vi "34970_CRISTALIZADOR Module.vi"(5 "Agilent 34970A":bool=TRUE, 6 "Freq(T)/Total":bool=TRUE, 7 "Command":T2, 8 "error in (no error)":errorcluster, 10 "Canales":T1={"CH PT100"=["201", "202", "205", "210"], "CH TcK"=["208"], "CH Qhz"=["208"]}, 11 "VISA Agilent 34970A":refnum<visa-resource-name>="COM42") -> (0 "error out":errorcluster, 1 "Qhz":dbl[](array[numeric]), 2 "TcK":dbl[](array[numeric]), 3 "PT100":dbl[](array[numeric]))   [LabVIEW 2017]
uses:
  34970_CRISTALIZADOR Module.ctl
  34970_Canales.ctl
  <instrlib>/Agilent 34970/Agilent 34970.lvlib
panel:
  # "Input Data"
  # "Output Data"
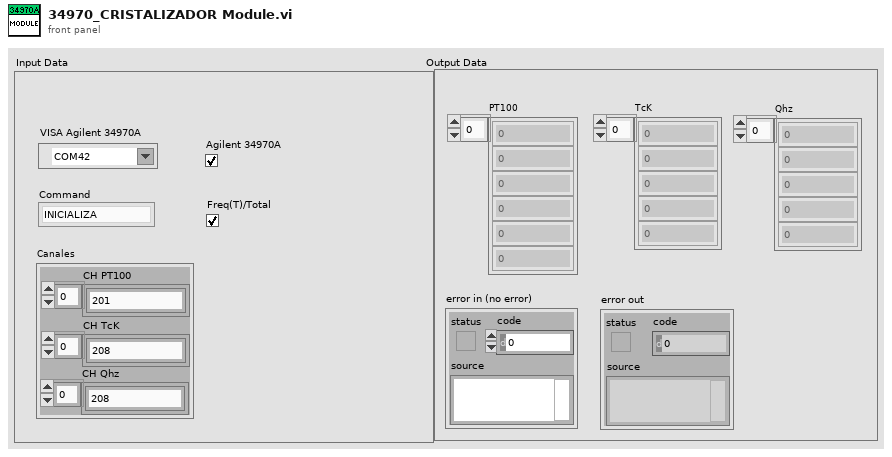
[diagram p1: front panel]
types:
  T1 = typedef "34970_Canales.ctl" = cluster{"CH PT100":string[], "CH TcK":string[], "CH Qhz":string[]}
  T2 = typedef "34970_CRISTALIZADOR Module.ctl" = enum16{"INICIALIZA", "CONFIGURA CANALES", "LECTURA PT100", "LECTURA TERMOPAR", "LECTURA CAUDAL", "LECTURA VOLTAJE", "LECTURA CORRIENTE", "SHUTDOWN"}
  T3 = cluster{"Timeout Value (10000)":u32, "Baud Rate (57600)":enum16{"1200", "2400", "4800", "9600", "19200", "38400", "57600", "115200"}, "Flow Control (1:XON/XOFF)":enum16{"None", "XON / XOFF", "RTS / CTS", "DTR / DSR"}}
  T4 = enum16{"Thermocouple", "Thermistor", "RTD", "4-Wire RTD", "Default (Last)"}
  T5 = enum16{"B", "E", "J", "K", "N", "R", "S", "T", "Default (Last)"}
  T6 = enum16{"100 mV", "1 V", "10 V", "100 V", "300 V", "Auto", "Minimum", "Maximum"}
  T7 = enum16{"4 1/2", "5 1/2", "6 1/2", "Least", "Highest", "Default"}
  T8 = enum16{"10 mA", "100 mA", "1 A", "Auto", "Minimum", "Maximum"}
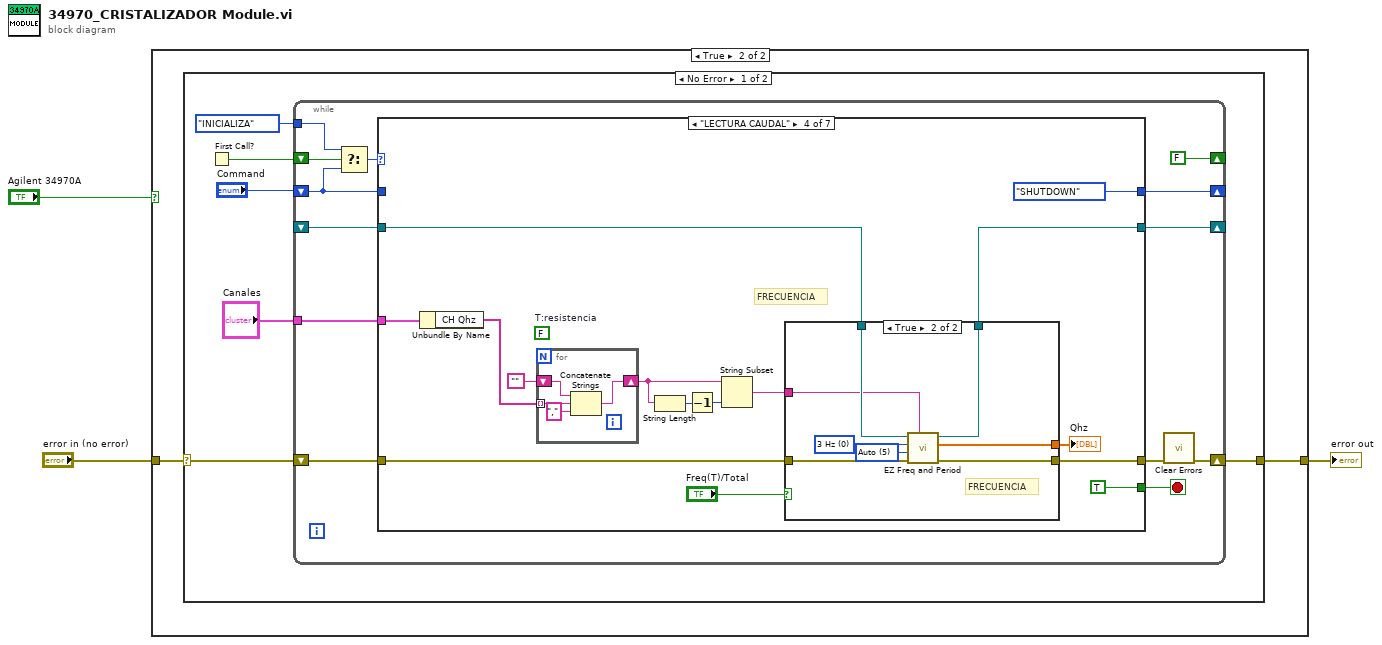
[diagram p0: block diagram]
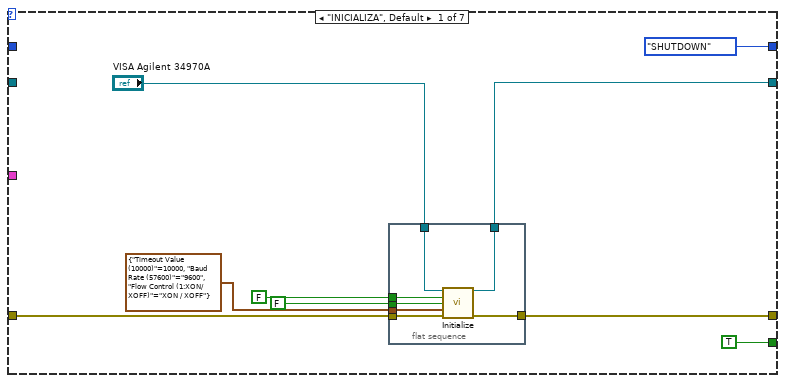
[diagram p3: hidden frame]
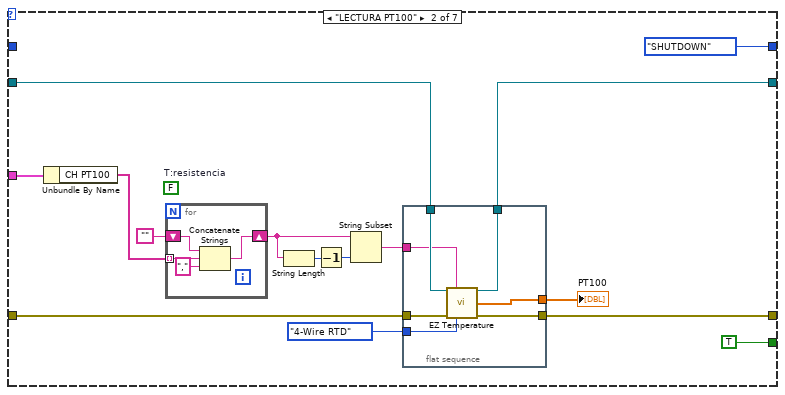
[diagram p4: hidden frame]
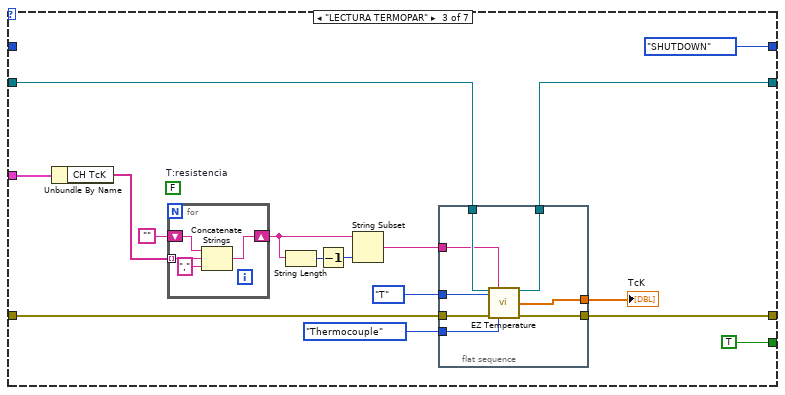
[diagram p5: hidden frame]
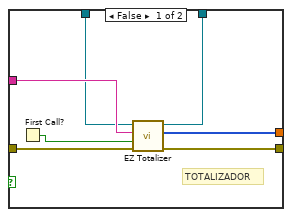
[diagram p6: hidden frame]
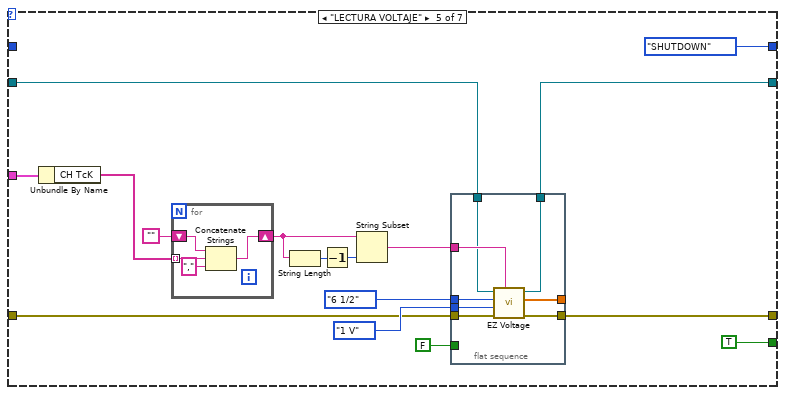
[diagram p7: hidden frame]
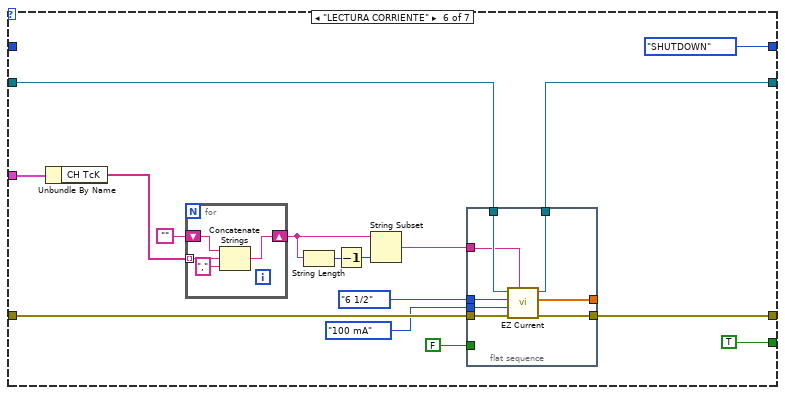
[diagram p8: hidden frame]
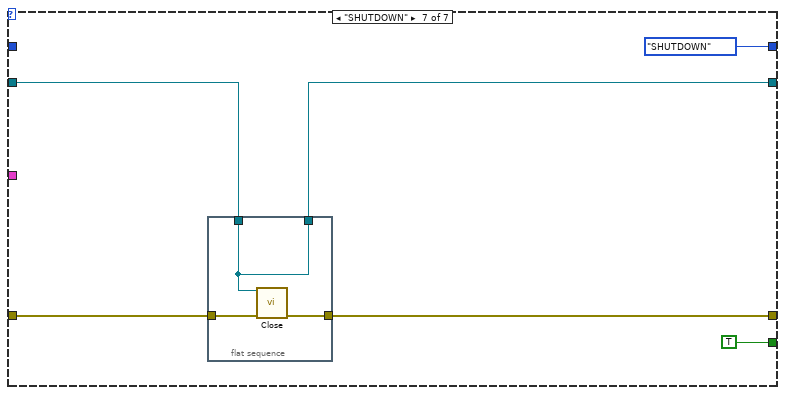
[diagram p9: hidden frame]
diagram:
  n1 = case shown="True" "Agilent 34970A" {
    tunnel: "error in (no error)" -> [w4 w6]
    tunnel: [w4 w5] -> w2
    frame False {
    }
    frame True {
      n2 = case shown="No Error" w6 {
        selector: w6 -> [w10 w195]
        tunnel: [w9 w195] -> w5
        frame No Error {
          n3 = First Call?() -> (First Call?: T/F=w12:bool)
          n4 = while {
            shift-right: [w19] -> _
            shift-left: "Command" -> [w20]
            shift-right: [w13] -> w9
            shift-left: w10 -> [w22]
            shift-right: [FALSE ("First Call?: T/F")] -> _
            shift-left: w12 -> [w25]
            tunnel: 34970_CRISTALIZADOR_Module."INICIALIZA" ("t") -> [w24]
            shift-right: [w17] -> _
            shift-left: _ -> [w18]
            tunnel: "Canales" -> [w15]
            stop <- w23 stop-if-true
            n5 = Select(t=w24, s=w25, f=w20) -> (s? t:f=w16:T2)
            n6 = case shown="\"LECTURA CAUDAL\"" w16 {
              tunnel: [TRUE TRUE TRUE TRUE TRUE TRUE TRUE] -> w23
              tunnel: w22 -> [w31 w53 w80 w107 w133 w163 w191]
              tunnel: w20 -> [_ _ _ _ _ _ _]
              tunnel: [34970_CRISTALIZADOR_Module."SHUTDOWN" ("t") 34970_CRISTALIZADOR_Module."SHUTDOWN" ("t") 34970_CRISTALIZADOR_Module."SHUTDOWN" ("t") 34970_CRISTALIZADOR_Module."SHUTDOWN" ("t") 34970_CRISTALIZADOR_Module."SHUTDOWN" ("t") 34970_CRISTALIZADOR_Module."SHUTDOWN" ("t") 34970_CRISTALIZADOR_Module."SHUTDOWN" ("t")] -> w19
              tunnel: [w30 w47 w74 w101 w142 w170 w190] -> w14
              tunnel: w18 -> [_ w54 w81 w108 w132 w162 w187]
              tunnel: [w29 w46 w73 w100 w143 w171 w186] -> w17
              tunnel: w15 -> [_ w44 w72 w99 w131 w159 _]
              frame "INICIALIZA", Default {
                n7 = flat-sequence {
                  tunnel: "VISA Agilent 34970A" -> [w40]
                  tunnel: w31 -> [w39]
                  tunnel: [w38] -> w30
                  tunnel: [w41] -> w29
                  tunnel: T3 {"Timeout Value (10000)"=10000, "Baud Rate (57600)"=enum."9600", "Flow Control (1:XON/XOFF)"=enum."XON / XOFF"} ("Serial Port Configuration") -> [w37]
                  tunnel: FALSE ("Reset (T: Reset)") -> [w36]
                  tunnel: FALSE ("ID Query (T: Check)") -> [w35]
                  frame #0 {
                    n8 = call <instrlib>:"Initialize.vi"("VISA Resource Name"=w40, "ID Query (T: Check)"=w35, "Reset (T: Reset)"=w36, "Serial Port Configuration"=w37, "error in (no error)"=w39) -> ("VISA Resource Name Out"=w41:refnum<visa-resource-name>, "error out"=w38:errorcluster)  [unwired: 9 in]
                  }
                }
              }
              frame "LECTURA PT100" {
                (unwired) FALSE  # T:resistencia
                n9 = Unbundle By Name(w44) -> ("CH PT100"=w43:string[])
                n10 = for {
                  tunnel: w43 -> [w66] mode=indexing
                  shift-right: [w65] -> w52
                  shift-left: "" -> [w67]
                  n11 = Concatenate Strings(w67, w66, "," ("string")) -> (w65:string)
                }
                n12 = String Length(string=w52) -> (length=w50:i32)
                n13 = Decrement(x=w50) -> (x-1=w51:i32)
                n14 = String Subset(string=w52, length (rest)=w51) -> (substring=w48:string)  [unwired: 1 in]
                n15 = flat-sequence {
                  tunnel: w54 -> [w63]
                  tunnel: w53 -> [w59]
                  tunnel: w48 -> [w57]
                  tunnel: [w61] -> w47
                  tunnel: [w62] -> w46
                  tunnel: [w60] -> w45
                  tunnel: T4."4-Wire RTD" ("Transducer Type (4:Def-Last)") -> [w58]
                  frame #0 {
                    n16 = call <instrlib>:"EZ Temperature.vi"("VISA Resource Name"=w63, "Scan List (empty)"=w57, "error in (no error)"=w59, "Transducer Type (4:Def-Last)"=w58) -> ("VISA Resource Name Out"=w62:refnum<visa-resource-name>, "Output Array"=w60:dbl[], "error out"=w61:errorcluster)  [unwired: 9 in]
                  }
                }
                "PT100" <- w45
              }
              frame "LECTURA TERMOPAR" {
                (unwired) FALSE  # T:resistencia
                n17 = Unbundle By Name(w72) -> ("CH TcK"=w71:string[])
                n18 = for {
                  tunnel: w71 -> [w94] mode=indexing
                  shift-right: [w93] -> w79
                  shift-left: "" -> [w95]
                  n19 = Concatenate Strings(w95, w94, "," ("string")) -> (w93:string)
                }
                n20 = String Length(string=w79) -> (length=w77:i32)
                n21 = Decrement(x=w77) -> (x-1=w78:i32)
                n22 = String Subset(string=w79, length (rest)=w78) -> (substring=w75:string)  [unwired: 1 in]
                n23 = flat-sequence {
                  tunnel: w81 -> [w91]
                  tunnel: w80 -> [w87]
                  tunnel: w75 -> [w85]
                  tunnel: [w89] -> w74
                  tunnel: [w90] -> w73
                  tunnel: [w88] -> w69
                  tunnel: T4."Thermocouple" ("Transducer Type (4:Def-Last)") -> [w86]
                  tunnel: T5."T" ("Thermocouple Type (8:Def-Last)") -> [w84]
                  frame #0 {
                    n24 = call <instrlib>:"EZ Temperature.vi"("VISA Resource Name"=w91, "Scan List (empty)"=w85, "Thermocouple Type (8:Def-Last)"=w84, "error in (no error)"=w87, "Transducer Type (4:Def-Last)"=w86) -> ("VISA Resource Name Out"=w90:refnum<visa-resource-name>, "Output Array"=w88:dbl[], "error out"=w89:errorcluster)  [unwired: 8 in]
                  }
                }
                "TcK" <- w69
              }
              frame "LECTURA CAUDAL" {
                (unwired) FALSE  # T:resistencia
                # "FRECUENCIA"
                n25 = Unbundle By Name(w99) -> ("CH Qhz"=w98:string[])
                n26 = for {
                  tunnel: w98 -> [w128] mode=indexing
                  shift-right: [w127] -> w106
                  shift-left: "" -> [w129]
                  n27 = Concatenate Strings(w129, w128, "," ("string")) -> (w127:string)
                }
                n28 = String Length(string=w106) -> (length=w104:i32)
                n29 = Decrement(x=w104) -> (x-1=w105:i32)
                n30 = String Subset(string=w106, length (rest)=w105) -> (substring=w102:string)  [unwired: 1 in]
                n31 = case shown="True" "Freq(T)/Total" {
                  tunnel: w108 -> [w114 w125]
                  tunnel: w107 -> [w117 w124]
                  tunnel: w102 -> [w116 w123]
                  tunnel: [w113 w122] -> w101
                  tunnel: [w115 w121] -> w100
                  tunnel: [w112 w120] -> w97
                  frame False {
                    # "TOTALIZADOR"
                    n32 = First Call?() -> (First Call?: T/F=w111:bool)
                    n33 = call <instrlib>:"EZ Totalizer.vi"("error in (no error)"=w117, "Read/R-Reset (F:Read)"=w111, "Scan List (empty)"=w116, "VISA Resource Name"=w114) -> ("error out"=w113:errorcluster, "Output Array"=w112:u32[], "VISA Resource Name Out"=w115:refnum<visa-resource-name>)  [unwired: 5 in]
                  }
                  frame True {
                    w118 = u16 5 items=["100 mV", "1 V", "10 V", "100 V", "300 V", "Auto", "Minimum", "Maximum"] ("Range (5:Auto)")
                    w119 = u16 0 items=["3 Hz", "20 Hz", "200 Hz", "MIN", "MAX"] ("Low Frequency (1: 20 Hz)")
                    # "FRECUENCIA"
                    n34 = call <instrlib>:"EZ Freq and Period.vi"("Scan List (empty)"=w123, "error in (no error)"=w124, "Range (5:Auto)"=w118, "Low Frequency (1: 20 Hz)"=w119, "VISA Resource Name"=w125) -> ("error out"=w122:errorcluster, "Output Array"=w120:dbl[], "VISA Resource Name Out"=w121:refnum<visa-resource-name>)  [unwired: 4 in]
                  }
                }
                "Qhz" <- w97
              }
              frame "LECTURA VOLTAJE" {
                n35 = Unbundle By Name(w131) -> ("CH TcK"=w130:string[])
                n36 = for {
                  tunnel: w130 -> [w156] mode=indexing
                  shift-right: [w155] -> w141
                  shift-left: "" -> [w157]
                  n37 = Concatenate Strings(w157, w156, "," ("string")) -> (w155:string)
                }
                n38 = String Length(string=w141) -> (length=w139:i32)
                n39 = Decrement(x=w139) -> (x-1=w140:i32)
                n40 = String Subset(string=w141, length (rest)=w140) -> (substring=w134:string)  [unwired: 1 in]
                n41 = flat-sequence {
                  tunnel: [w146] -> w143
                  tunnel: [w150] -> w142
                  tunnel: FALSE ("AC/DC (F:DC)") -> [_]
                  tunnel: T7."6 1/2" ("Resolution (5:Default)") -> [w147]
                  tunnel: T6."1 V" ("Range (5:Auto)") -> [w148]
                  tunnel: w134 -> [w153]
                  tunnel: w133 -> [w149]
                  tunnel: w132 -> [w152]
                  tunnel: [w151] -> _
                  frame #0 {
                    n42 = call <instrlib>:"EZ Voltage.vi"("Scan List (empty)"=w153, "error in (no error)"=w149, "Range (5:Auto)"=w148, "Resolution (5:Default)"=w147, "VISA Resource Name"=w152) -> ("error out"=w150:errorcluster, "Output Array"=w151:dbl[], "VISA Resource Name Out"=w146:refnum<visa-resource-name>)  [unwired: 4 in]
                  }
                }
              }
              frame "LECTURA CORRIENTE" {
                n43 = Unbundle By Name(w159) -> ("CH TcK"=w158:string[])
                n44 = for {
                  tunnel: w158 -> [w184] mode=indexing
                  shift-right: [w183] -> w169
                  shift-left: "" -> [w185]
                  n45 = Concatenate Strings(w185, w184, "," ("string")) -> (w183:string)
                }
                n46 = String Length(string=w169) -> (length=w167:i32)
                n47 = Decrement(x=w167) -> (x-1=w168:i32)
                n48 = String Subset(string=w169, length (rest)=w168) -> (substring=w164:string)  [unwired: 1 in]
                n49 = flat-sequence {
                  tunnel: [w180] -> w171
                  tunnel: [w178] -> w170
                  tunnel: FALSE ("AC/DC (F:DC)") -> [_]
                  tunnel: w164 -> [w174]
                  tunnel: w163 -> [w179]
                  tunnel: w162 -> [w181]
                  tunnel: T7."6 1/2" ("Resolution (3:Least)") -> [w176]
                  tunnel: T8."100 mA" ("Range (3:Auto)") -> [w175]
                  tunnel: [w177] -> _
                  frame #0 {
                    n50 = call <instrlib>:"EZ Current.vi"("Scan List (empty)"=w174, "error in (no error)"=w179, "Range (3:Auto)"=w175, "Resolution (3:Least)"=w176, "VISA Resource Name"=w181) -> ("error out"=w178:errorcluster, "Output Array"=w177:dbl[], "VISA Resource Name Out"=w180:refnum<visa-resource-name>)  [unwired: 4 in]
                  }
                }
              }
              frame "SHUTDOWN" {
                n51 = flat-sequence {
                  tunnel: w191 -> [w193]
                  tunnel: [w192] -> w190
                  tunnel: [w194] -> w186
                  tunnel: w187 -> [w194]
                  frame #0 {
                    n52 = call <instrlib>:"Close.vi"("VISA Resource Name"=w194, "error in (no error)"=w193) -> ("error out"=w192:errorcluster)  [unwired: 13 in]
                  }
                }
              }
            }
            n53 = call <vilib>:"Clear Errors.vi"("error in (no error)"=w14) -> ("error out"=w13:errorcluster)  [unwired: 5 in, 1 out]
          }
        }
        frame Error {
        }
      }
    }
  }
  "error out" <- w2
